vi "Create_directory_and_files.vi"(8 "error in":errorcluster, 9 "NE":string, 10 "DE":path, 11 "ClusterIn":T1={"Simulation?"=FALSE, "ChanConfigs"=[], "Essay Config"={"HoleDiam"=1.4, "MeanLineDiam"=5.0, "IncF"=0.2, "ElastMod"=207.0, "PoissonMod"=0.3, "RosType"=enum."Tipo A", "Método de análise"=enum."Simplificado 2008", "Pfinal"=0.3, "AStop"=TRUE}, "Directory"=path "", "EssayName"="", "RawFile"=refnum, "InfoFile"=refnum, "DataFile"=refnum, "task"="", "qRecord"=refnum, "qProcess"=refnum} {"ChanConfigs"."GF" min=0.1 max=10.0; "ChanConfigs"."Canal" min=1 max=8}) -> (0 "error out":errorcluster, 3 "ClusterOut":T1={"Simulation?"=FALSE, "ChanConfigs"=[], "Essay Config"={"HoleDiam"=1.4, "MeanLineDiam"=5.0, "IncF"=0.2, "ElastMod"=207.0, "PoissonMod"=0.3, "RosType"=enum."Tipo A", "Método de análise"=enum."Simplificado 2008", "Pfinal"=0.3, "AStop"=TRUE}, "Directory"=path "", "EssayName"="", "RawFile"=refnum, "InfoFile"=refnum, "DataFile"=refnum, "task"="", "qRecord"=refnum, "qProcess"=refnum} {"ChanConfigs"."GF" min=0.1 max=10.0; "ChanConfigs"."Canal" min=1 max=8})   [LabVIEW 2016]
uses:
  MainFGV/cluster_main_FGV.ctl
  Config/Channel_config.ctl
  Config/essay_config.ctl
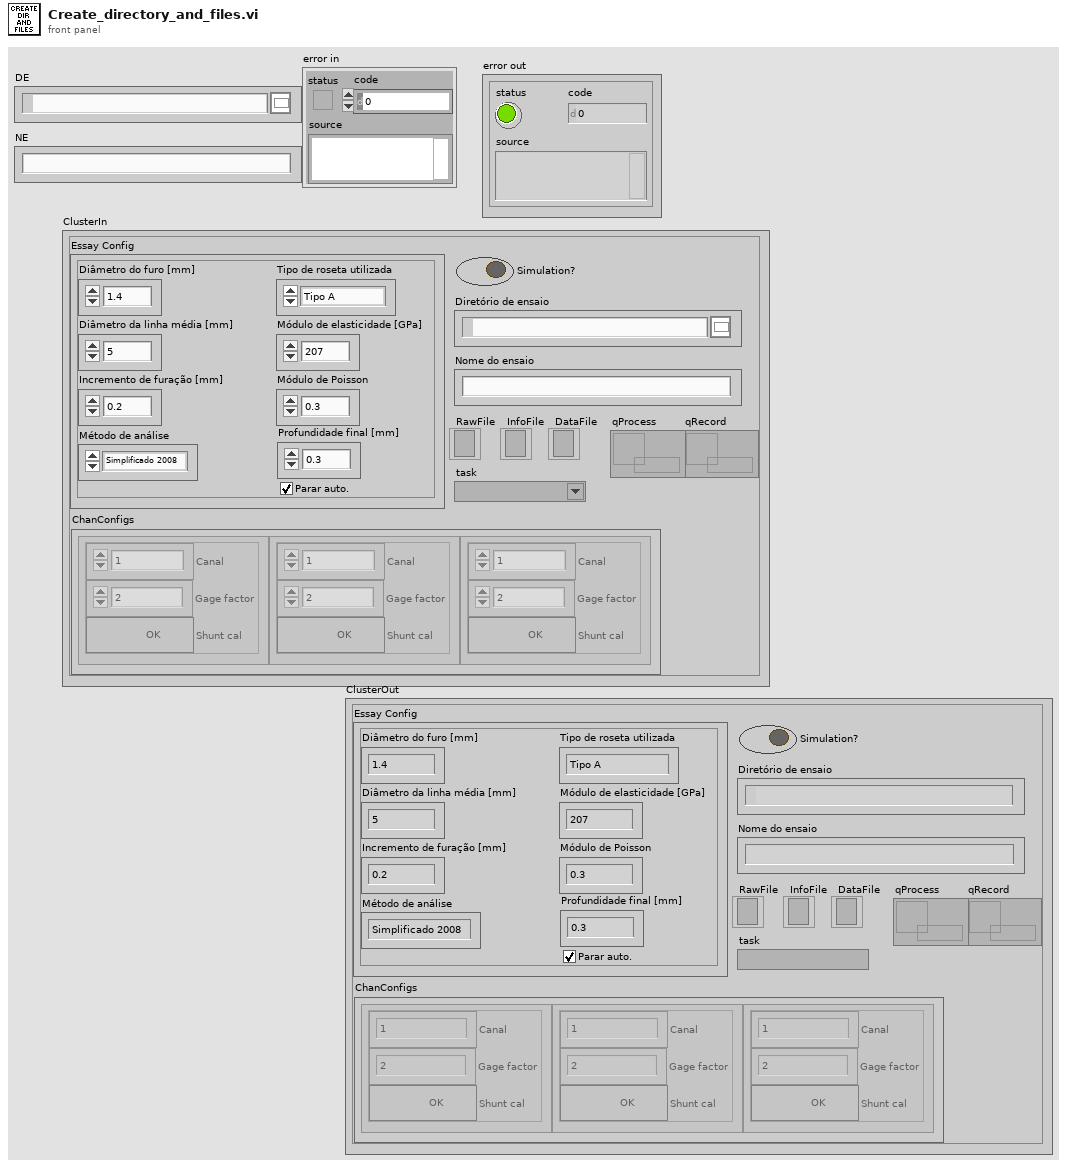
[diagram p1: front panel]
types:
  T1 = typedef "cluster_main_FGV.ctl" = cluster{"Simulation?":bool, "ChanConfigs":T2[], "Essay Config":T3, "Directory":path, "EssayName":string, "RawFile":refnum<file>, "InfoFile":refnum<file>, "DataFile":refnum<file>, "task":refnum<k21>, "qRecord":refnum<queue>, "qProcess":refnum<queue>}
  T2 = typedef "Channel_config.ctl" = cluster{"Canal":i32, "GF":dbl, "SC":bool}
  T3 = typedef "essay_config.ctl" = cluster{"HoleDiam":dbl, "MeanLineDiam":dbl, "IncF":dbl, "ElastMod":dbl, "PoissonMod":dbl, "RosType":enum16{"Tipo A", "Tipo B", "Tipo C"}, "Método de análise":enum16{"Não uniforme 2013", "Simplificado 2013", "Simplificado 2008"}, "Pfinal":dbl, "AStop":bool}
  T4 = enum16{"open", "replace", "create", "open or create", "replace or create", "replace or create with confirmation"}
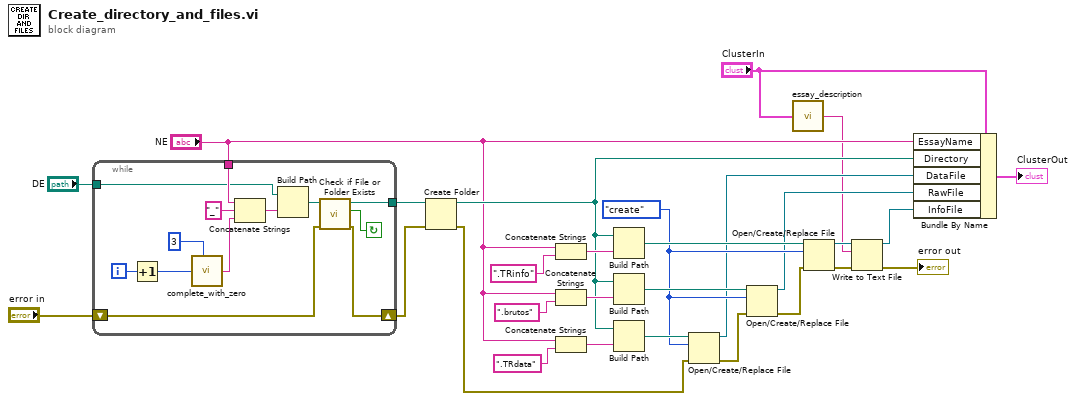
[diagram p0: block diagram]
diagram:
  w6 = T4."create" ("operation (0:open)")
  n1 = while {
    tunnel: "DE" -> [w34]
    tunnel: "NE" -> [w38]
    shift-right: [w30] -> w25
    shift-left: "error in" -> [w31]
    tunnel: [w29] -> w26
    i -> [w41]
    stop <- w32 continue-if-true
    n2 = Increment(x=w41) -> (x+1=w39:i32)
    n3 = call "complete_with_zero.vi"("#Chars"=3, "Number"=w39) -> ("StringOut"=w37:string)  [unwired: 3 in]
    n4 = Concatenate Strings(w38, "_" ("string"), w37) -> (w35:string)
    n5 = Build Path(base path=w34, name or relative path=w35) -> (appended path=w33:path)
    n6 = call <vilib>:"Check if File or Folder Exists.vi"("error in (no error)"=w31, "path"=w33) -> ("error out"=w30:errorcluster, "file or folder exists?"=w32:bool, "dup path"=w29:path)  [unwired: 7 in]
  }
  n7 = Create Folder(path (use dialog)=w26, error in=w25) -> (created path=w14:path, error out=w16:errorcluster)  [unwired: 1 in, 1 out]
  n8 = Concatenate Strings("NE", ".TRinfo" ("string")) -> (w15:string)
  n9 = Concatenate Strings("NE", ".brutos" ("string")) -> (w18:string)
  n10 = Concatenate Strings("NE", ".TRdata" ("string")) -> (w21:string)
  n11 = Build Path(base path=w14, name or relative path=w15) -> (appended path=w11:path)
  n12 = Build Path(base path=w14, name or relative path=w18) -> (appended path=w19:path)
  n13 = Build Path(base path=w14, name or relative path=w21) -> (appended path=w22:path)
  n14 = Open/Create/Replace File(file path (use dialog)=w22, error in=w16, operation (0:open)=w6) -> (refnum out=w5:refnum<file>, error out=w23:errorcluster)  [unwired: 3 in, 1 out]
  n15 = Open/Create/Replace File(file path (use dialog)=w19, error in=w23, operation (0:open)=w6) -> (refnum out=w4:refnum<file>, error out=w10:errorcluster)  [unwired: 3 in, 1 out]
  n16 = call "essay_description.vi"("cluster_main_FGV"="ClusterIn") -> ("EssayDescription"=w1:string)
  n17 = Open/Create/Replace File(file path (use dialog)=w11, error in=w10, operation (0:open)=w6) -> (refnum out=w8:refnum<file>, error out=w9:errorcluster)  [unwired: 3 in, 1 out]
  n18 = Write to Text File(file (use dialog)=w8, text=w1, error in=w9) -> (refnum out=w3:refnum<file>, error out=→"error out":errorcluster)  [unwired: 1 in, 1 out]
  n19 = Bundle By Name(cluster="ClusterIn", "EssayName"="NE", "Directory"=w14, "DataFile"=w5, "RawFile"=w4, "InfoFile"=w3) -> (→"ClusterOut":T1)
